vi "Write Roles.vi"(8 "error in (no error)":errorcluster, 10 "Roles":T1, 11 "NormalDefensivePlay in":refnum<class "NormalDefensivePlay.lvclass">) -> (0 "error out":errorcluster, 3 "NormalDefensivePlay out":refnum<class "NormalDefensivePlay.lvclass">)   [LabVIEW 2023, in "NormalDefensivePlay.lvclass"]
uses:
  NormalDefensivePlay.lvclass
  DefenderAreaRole_class/DefenderAreaRole.lvclass
  NormalDefensivePlay.lvclass/NormalDefensivePlay.ctl
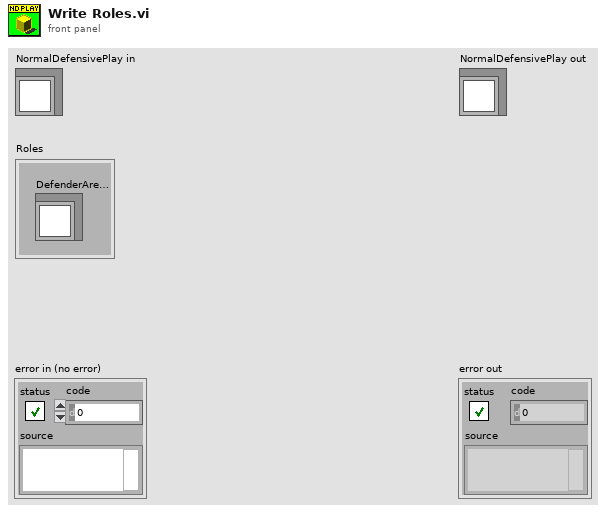
[diagram p1: front panel]
types:
  T1 = cluster{"DefenderAreaRole":refnum<class "DefenderAreaRole.lvclass">}
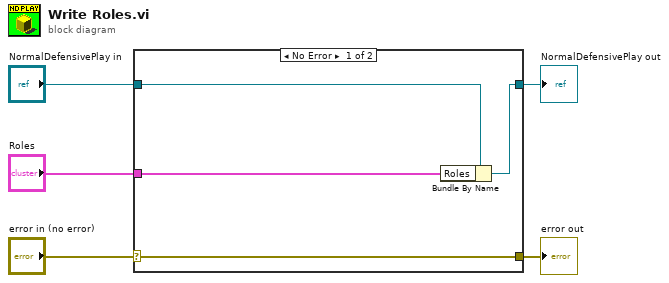
[diagram p0: block diagram]
diagram:
  n1 = case shown="No Error" "error in (no error)" {
    selector: "error in (no error)" -> [w9 w10]
    tunnel: [w9 w10] -> w4
    tunnel: [w7 w11] -> w2
    tunnel: "NormalDefensivePlay in" -> [w8 w11]
    tunnel: "Roles" -> [w6 _]
    frame No Error {
      n2 = Bundle By Name(cluster=w8, "Roles"=w6) -> (w7:refnum<class "NormalDefensivePlay.lvclass">)
    }
    frame Error {
    }
  }
  "error out" <- w4
  "NormalDefensivePlay out" <- w2
